vi "Rio_Collect_Kicker (DONE).vi"(8 "error in (no error)":errorcluster, 11 "Kicker Collection \nPosition":dbl) -> (0 "error out":errorcluster, 3 "Boolean":bool)   [LabVIEW 2017]
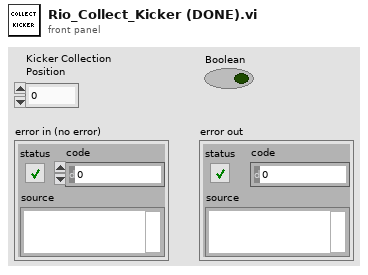
[diagram p1: front panel]
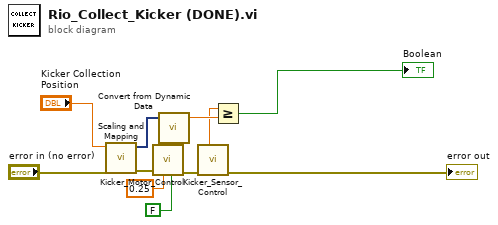
[diagram p0: block diagram]
diagram:
  n1 = call "Scaling and Mapping"("error in (no error)"="error in (no error)", "Signals"="Kicker Collection \nPosition") -> ("error out"=w9:errorcluster, "Scaled Signals"=w10:dynamicdata)  [unwired: 8 in]
  n2 = call "Kicker_Motor_Control.vi"("Motor Dir (T/F = U/D)"=FALSE ("Motor Dir"), "Duty Cycle"=0.25 ("Motor Speed"), "error in"=w9) -> ("error out"=w1:errorcluster)  [unwired: 8 in]
  n3 = call "Convert from Dynamic Data"("Dynamic Data Type"=w10) -> ("Scalar"=w11:dbl)  [unwired: 3 in]
  n4 = call "Kicker_Sensor_Control.vi"("error in"=w1) -> ("error out"=→"error out":errorcluster, "Pot Output"=w2:dbl)  [unwired: 9 in]
  n5 = Greater Or Equal?(x=w2, y=w11) -> (x >= y?=→"Boolean":bool)
